vi "Read C declarations into text ring.vi"() -> ()   [LabVIEW 2009, in "HighFinesse WS5.lvlib"]
uses:
  HighFinesse WS5.lvlib
panel:
  in  "Ring":i16(ring) items=["ErrNoValue"=0, "ErrNoSignal"=-1, "ErrNoPulse"=-8, "ErrBadSignal"=-2, "ErrLowSignal"=-3, "ErrBigSignal"=-4, "ErrWlmMissing"=-5, "ErrNotAvailable"=-6, "InfNothingChanged"=-7, "ErrDiv0"=-13, "ErrOutOfRange"=-14, "ErrUnitNotAvailable"=-15, "ErrTemperature"=-1000, "ErrTempNotAvailable"=-996, "ErrTempWlmMissing"=-995, "ErrDistance"=13824, "ErrDistanceNotAvailable"=13830, "ErrDistanceWlmMissing"=13829]
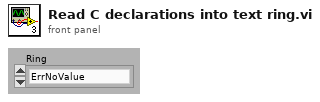
[diagram p1: front panel]
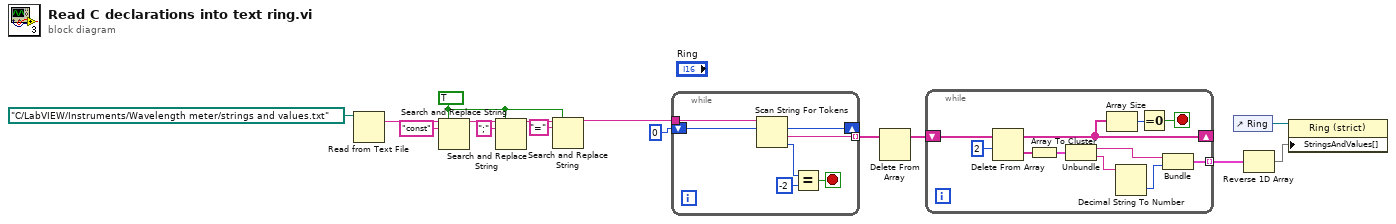
[diagram p0: block diagram]
diagram:
  w6 = TRUE
  n1 = Read from Text File(file (use dialog)=path "C:/LabVIEW/Instruments/Wavelength meter/strings and values.txt") -> (text=w10:string)  [unwired: 1 in, 5 out]
  n2 = Search and Replace String(replace all?=w6, input string=w10, search string="const") -> (result string=w12:string)  [unwired: 1 in, 7 out]
  n3 = Search and Replace String(replace all?=w6, input string=w12, search string=";") -> (result string=w9:string)  [unwired: 1 in, 7 out]
  n4 = Search and Replace String(replace all?=w6, input string=w9, search string="=") -> (result string=w7:string)  [unwired: 1 in, 7 out]
  n5 = while {
    shift-right: [w22] -> _
    shift-left: 0 ("offset past token") -> [w18]
    tunnel: [w17] -> w5 mode=indexing
    tunnel: w7 -> [w16]
    stop <- w19 stop-if-true
    n6 = Scan String For Tokens(8:w18, 9:w16) -> (0:w21:i32, 1:w17:string, 2:w22:i32)  [unwired: 5 out]
    n7 = Equal?(x=w21, y=-2) -> (x = y?=w19:bool)
  }
  n8 = Delete From Array(array=w5) -> (array with subset deleted=w4:string[])  [unwired: 2 in, 1 out]
  n9 = while {
    shift-right: [w29] -> _
    shift-left: w4 -> [w32]
    tunnel: [w23] -> w2 mode=indexing
    stop <- w30 stop-if-true
    n10 = Delete From Array(array=w32, length=2) -> (deleted portion=w28:string[], array with subset deleted=w29:string[])  [unwired: 1 in]
    n11 = Array To Cluster(array=w28) -> (cluster=w27:cluster{"[0]":string, "[1]":string})
    n12 = Unbundle(w27) -> ("[0]"=w24:string, "[1]"=w26:string)
    n13 = Array Size(array=w29) -> (size(s)=w31:i32)
    n14 = Decimal String To Number(string=w26) -> (number=w25:i32)  [unwired: 3 out]
    n15 = Equal To 0?(x=w31) -> (x = 0?=w30:bool)
    n16 = Bundle("[0]"=w24, w25) -> (w23:cluster{"[0]":string, i32})  [unwired: 1 out]
  }
  n17 = control-ref of="Ring"() -> (w3:refnum<vi>)
  n18 = Reverse 1D Array(array=w2) -> (reversed array=w1:cluster{"[0]":string, i32}[])
  n19 = property class="Ring (strict)"(reference=w3, "StringsAndValues[]"=w1) -> ()  [unwired: 1 in, 2 out]
